vi "Bundler_Selected Element.vi"(7 "Action":T1=enum."Bundler Insert", 8 "error in (no error)":errorcluster, 11 "Affected Items":T2) -> (0 "error out":errorcluster, 1 "Selected Element Name":string, 2 "index of element":i32, 3 "Selected Element Term Refnum":refnum<vi>, 4 "last element":bool, 5 "Display String":string, 6 "first element":bool)   [LabVIEW 2023]
uses:
  top/BundleMagic.ctl
  controls/action enum.ctl
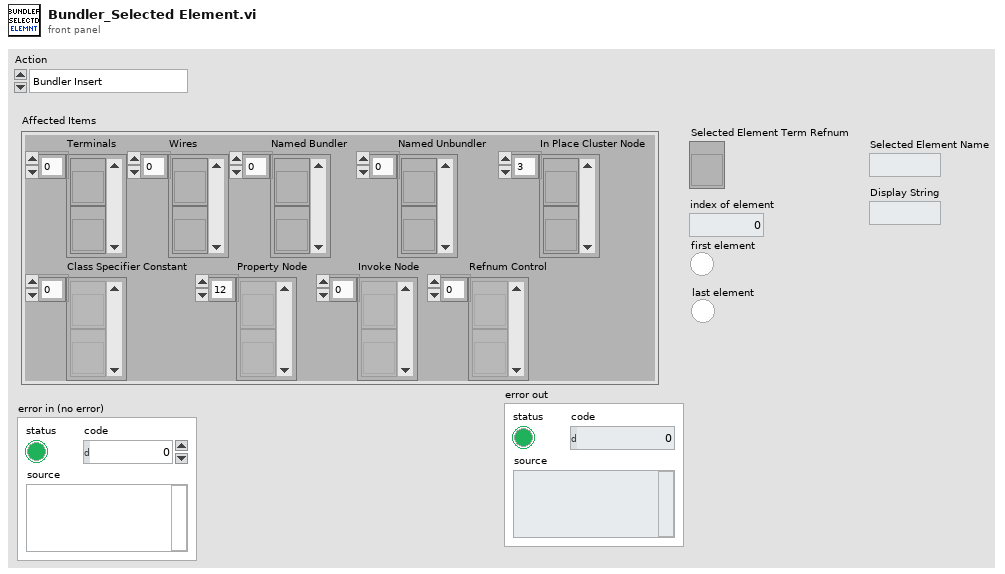
[diagram p1: front panel]
types:
  T1 = typedef "action enum.ctl" = enum16{"[NONE]", "Wire Bundle", "Wire Unbundle", "Terminal Unbundle", "Terminal Bundle", "Bundler Move Up", "Bundler Move Down", "Bundler Insert", "Bundler Remove", "Bundler Remove Unwired", "Bundler Rearrange", "In Place Insert", "In Place Remove", "In Place Remove Unwired", "In Place Rearrange", "Wire Properties", "Wire Method", "Terminal Properties", "Terminal Method", "Property Move Up", "Property Move Down", "Properties Insert", "Properties Remove", "Properties Remove Unwired", "Properties Rearrange", "Method Change", "Class For Constant", "Class For Control", "Class For Node", "Class Name to Clipboard"}
  T2 = typedef "BundleMagic.ctl" = cluster{"Terminals":refnum<vi>[], "Wires":refnum<vi>[], "Named Bundler":refnum<vi>[], "Named Unbundler":refnum<vi>[], "In Place Cluster Node":refnum<vi>[], "Class Specifier Constant":refnum<vi>[], "Property Node":refnum<vi>[], "Invoke Node":refnum<vi>[], "Refnum Control":refnum<vi>[]}
  T3 = enum16{"Named Bundler", "Named Unbundler", "In Place", "None"}
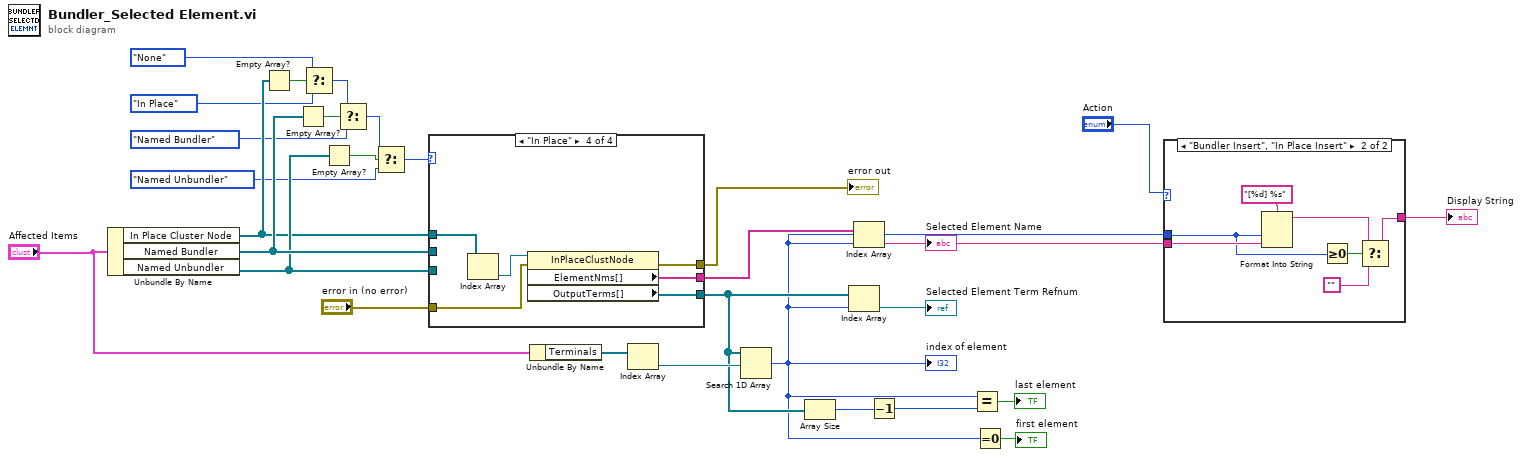
[diagram p0: block diagram]
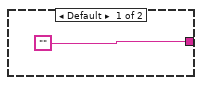
[diagram p2: hidden frame]
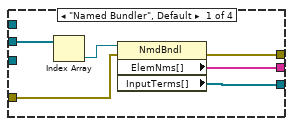
[diagram p3: hidden frame]
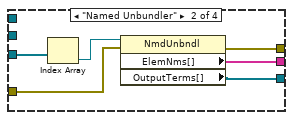
[diagram p4: hidden frame]
diagram:
  n1 = Unbundle By Name("Affected Items") -> ("In Place Cluster Node"=w15:refnum<vi>[], "Named Bundler"=w18:refnum<vi>[], "Named Unbundler"=w17:refnum<vi>[])
  n2 = Empty Array?(array=w15) -> (empty?=w16:bool)
  n3 = Empty Array?(array=w18) -> (empty?=w29:bool)
  n4 = Select(t=T3."None" ("Bundler Type"), s=w16, f=T3."In Place" ("Bundler Type")) -> (s? t:f=w10:T3)
  n5 = Empty Array?(array=w17) -> (empty?=w23:bool)
  n6 = Select(t=w10, s=w29, f=T3."Named Bundler" ("Bundler Type")) -> (s? t:f=w22:T3)
  n7 = Select(t=w22, s=w23, f=T3."Named Unbundler" ("Bundler Type")) -> (s? t:f=w11:T3)
  n8 = case shown="\"In Place\"" w11 {
    tunnel: w17 -> [_ w41 _ _]
    tunnel: w18 -> [w35 _ _ _]
    tunnel: [w33 w39 _ w48] -> w25
    tunnel: [w32 w38 _ w47] -> w9
    tunnel: w15 -> [_ _ _ w46]
    tunnel: "error in (no error)" -> [w31 w37 w42 w43]
    tunnel: [w30 w36 w42 w44] -> w1
    frame "Named Bundler", Default {
      n9 = Index Array(array=w35) -> (element=w34:refnum<vi>)  [unwired: 1 in]
      n10 = property class="NmdBndl"(reference=w34, error in=w31) -> (error out=w30:errorcluster, "ElemNms[]"=w33:string[], "InputTerms[]"=w32:refnum<vi>[])  [unwired: 1 out]
    }
    frame "Named Unbundler" {
      n11 = Index Array(array=w41) -> (element=w40:refnum<vi>)  [unwired: 1 in]
      n12 = property class="NmdUnbndl"(reference=w40, error in=w37) -> (error out=w36:errorcluster, "ElemNms[]"=w39:string[], "OutputTerms[]"=w38:refnum<vi>[])  [unwired: 1 out]
    }
    frame "None" {
    }
    frame "In Place" {
      n13 = Index Array(array=w46) -> (element=w45:refnum<vi>)  [unwired: 1 in]
      n14 = property class="InPlaceClustNode"(reference=w45, error in=w43) -> (error out=w44:errorcluster, "ElementNms[]"=w48:string[], "OutputTerms[]"=w47:refnum<vi>[])  [unwired: 1 out]
    }
  }
  "error out" <- w1
  n15 = Unbundle By Name("Affected Items") -> ("Terminals"=w27:refnum<vi>[])
  n16 = Index Array(array=w27) -> (element=w26:refnum<vi>)  [unwired: 1 in]
  n17 = Search 1D Array(1D array=w9, element=w26) -> (index of element=w4:i32)  [unwired: 1 in]
  "index of element" <- w4
  n18 = Array Size(array=w9) -> (size(s)=w8:i32)
  n19 = Index Array(array=w9, index=w4) -> (element=→"Selected Element Term Refnum":refnum<vi>)
  n20 = Index Array(array=w25, index=w4) -> (element=w3:string)
  "Selected Element Name" <- w3
  n21 = Decrement(x=w8) -> (x-1=w7:i32)
  n22 = Equal?(x=w4, y=w7) -> (x = y?=→"last element":bool)
  n23 = Equal To 0?(x=w4) -> (x = 0?=→"first element":bool)
  n24 = case shown="\"Bundler Insert\", \"In Place Insert\"" "Action" {
    tunnel: ["" w50] -> w20
    tunnel: w4 -> [_ w53]
    tunnel: w3 -> [_ w55]
    frame Default {
    }
    frame "Bundler Insert", "In Place Insert" {
      n25 = Format Into String(format string="[%d] %s", w53, w55) -> (resulting string=w51:string)  [unwired: 2 in, 1 out]
      n26 = Greater Or Equal To 0?(x=w53) -> (x >= 0?=w54:bool)
      n27 = Select(t=w51, s=w54, f="") -> (s? t:f=w50:string)
    }
  }
  "Display String" <- w20
